vi "Handle Messages.vi"(8 "error in (no error)":errorcluster, 9 "Message Data":variant, 10 "Message":string, 11 "Coffee Shop In":refnum<class "Coffee Shop.lvclass">) -> (0 "error out":errorcluster, 3 "Coffee Shop Out":refnum<class "Coffee Shop.lvclass">)   [LabVIEW 2020, in "Coffee Shop.lvclass"]
uses:
  Coffee Shop.lvclass
  C:/Program Files (x86)/National Instruments/LabVIEW 2020/vi.lib/Astemes/Triarc Framework/Application/Application.lvclass
  C:/Program Files (x86)/National Instruments/LabVIEW 2020/vi.lib/Astemes/Triarc Framework/Process/Process.lvclass
  People/Person/Person.lvclass
  Public/Roles.ctl
  <vilib>/Astemes/Triarc Framework/Process/Process.lvclass/Process.ctl
  <vilib>/Astemes/Triarc Framework/Application/Application.lvclass/Application.ctl
  Coffee Shop.lvclass/Coffee Shop.ctl
  People/Process Job/Job Handler.lvclass
  People/Workers/Cashier/Cashier.lvclass
  C:/Git/astemes-triarc-examples/source/Coffee Shop/Processes/People/Workers/Worker/Worker.lvclass
  People/Customers/Customer/Customer.lvclass
  People/Workers/Barista/Barista.lvclass
  <vilib>/Astemes/Triarc Framework/View/View.lvclass
  <vilib>/Astemes/Triarc Framework/View/View.lvclass/View.ctl
  <vilib>/Astemes/Triarc Framework/Application/Private/Add Process to Map.vi
  <vilib>/Astemes/Triarc Framework/Application/Private/Throw Error If Process Already in App.vi
  <vilib>/Astemes/Triarc Framework/Process/Protected/Messaging/Send Message.vi
  <vilib>/Astemes/Triarc Framework/Process/Public/Lifecycle/Get Lifecycle State.vi
  <vilib>/Astemes/Triarc Framework/Process/Protected/SubVIs/Set Context.vi
  <vilib>/Astemes/Triarc Framework/Process/Stop.vi
  <vilib>/Astemes/Triarc Framework/Application/Private/Remove Process from Map.vi
  <vilib>/Astemes/Triarc Framework/Process/Private/SubVIs/Handle Debug Data.vi
  <vilib>/Astemes/Triarc Framework/Application/Private/Retrieve Process from App.vi
  <vilib>/Astemes/Triarc Framework/Application/Private/Parse Process Name.vi
  <vilib>/Astemes/Triarc Framework/Application/Private/Get Process from Map.vi
  <vilib>/Astemes/Triarc Framework/View/Public/Get View VI Reference.vi
  <vilib>/Utility/error.llb/Clear Errors.vi
  <vilib>/Astemes/Triarc Framework/Process/Public/Lifecycle/Leave Process Loop.vi
  <vilib>/Astemes/Triarc Framework/Process/Private/SubVIs/Wait for finish.vi
  <vilib>/Astemes/Triarc Framework/Process/Private/SubVIs/Set Lifecycle State.vi
  <vilib>/Astemes/Triarc Framework/Logging/Log Debug.vi
  <vilib>/AdvancedString/1D String Array to Delimited String.vi
  <vilib>/Utility/High Resolution Relative Seconds.vi
  <vilib>/Astemes/Triarc Framework/Process/Protected/Messaging/Request Message.vi
  <vilib>/AdvancedString/Delimited String to 1D String Array.vi
  <vilib>/Astemes/Triarc Framework/Process/Private/SubVIs/Enqueue Request Message.vi
  <vilib>/Astemes/Triarc Framework/Application/Application.lvclass
  <vilib>/Utility/error.llb/Error Cluster From Error Code.vi
  <vilib>/Astemes/Triarc Framework/Process/Private/SubVIs/Wait for Response Message.vi
  <vilib>/Astemes/Triarc Framework/Process/Process.lvclass
  People/Workers/Worker/Worker.lvclass
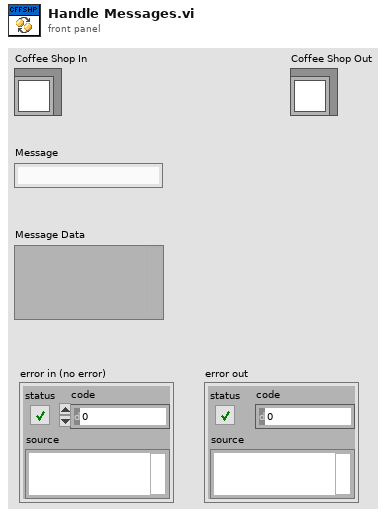
[diagram p1: front panel]
types:
  T1 = typedef "Coffee Shop.lvclass/Roles.ctl" = enum16{"Customer", "Barista", "Cashier"}
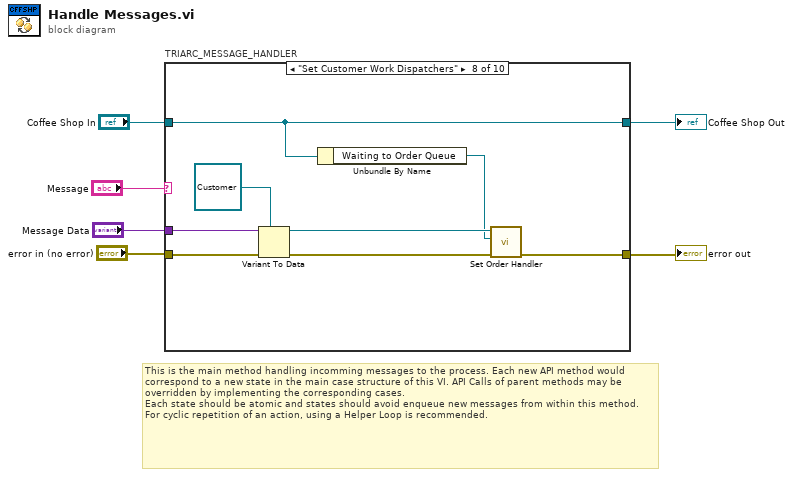
[diagram p0: block diagram]
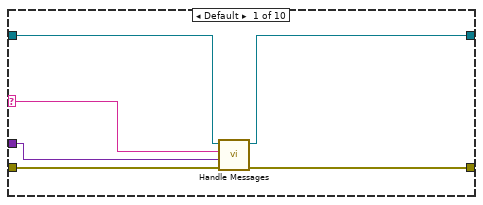
[diagram p2: hidden frame]
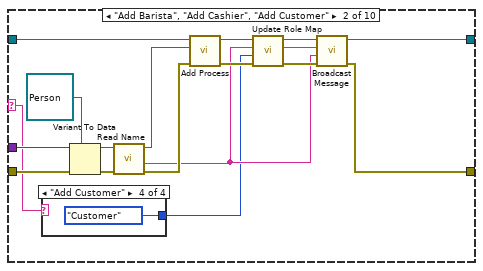
[diagram p3: hidden frame]
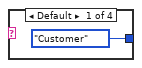
[diagram p4: hidden frame]
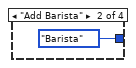
[diagram p5: hidden frame]
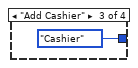
[diagram p6: hidden frame]
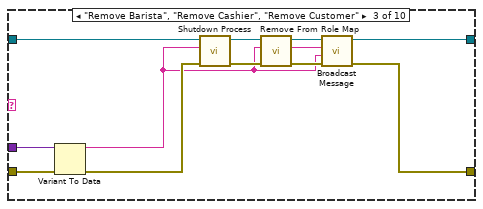
[diagram p7: hidden frame]
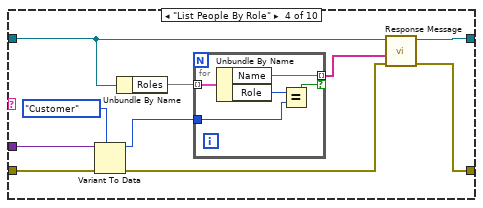
[diagram p8: hidden frame]
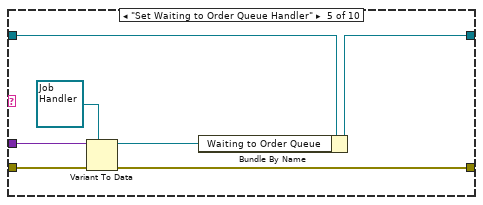
[diagram p9: hidden frame]
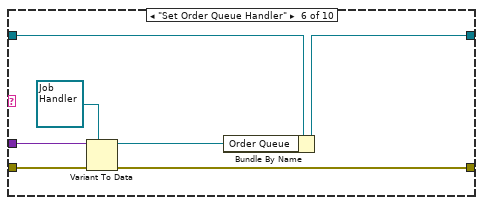
[diagram p10: hidden frame]
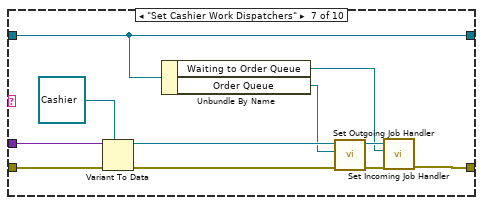
[diagram p11: hidden frame]
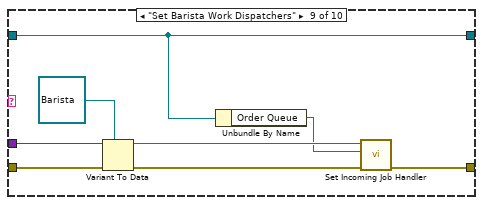
[diagram p12: hidden frame]
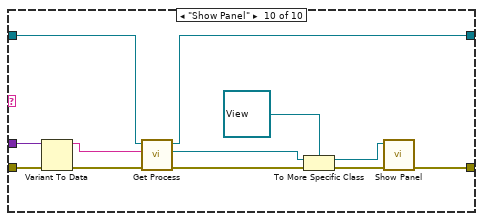
[diagram p13: hidden frame]
diagram:
  # "This is the main method handling incomming messages to the process. Each new API method would correspond to a new state in the main case structure of this VI. API Calls of parent methods may be overridden by implementing the corresponding cases.\nEach state should be atomic and states should avoid enqueue new messages from within this method. For cyclic repetition of an action, using a Helper Loop is recommended."
  n1 = case "TRIARC_MESSAGE_HANDLER" shown="\"Set Customer Work Dispatchers\"" "Message" {
    selector: "Message" -> [w10 w15 _ _ _ _ _ _ _ _]
    tunnel: "error in (no error)" -> [w9 w29 w46 w56 w68 w75 w86 w94 w102 w114]
    tunnel: "Coffee Shop In" -> [w12 w27 w44 w48 w67 w74 w83 w91 w99 w105]
    tunnel: "Message Data" -> [w11 w30 w45 w54 w64 w71 w84 w92 w100 w103]
    tunnel: [w8 w14 w41 w50 w66 w73 w80 w87 w97 w110] -> w2
    tunnel: [w7 w24 w40 w49 w63 w70 w83 w91 w99 w106] -> w1
    frame Default {
      n2 = call-parent "Handle Messages.vi"("error in (no error)"=w9, "Message Data"=w11, "Message"=w10, "Application In"=w12) -> ("error out"=w8:errorcluster, "Application Out"=w7:refnum<class "Coffee Shop.lvclass">)  [unwired: 6 in]
    }
    frame "Add Barista", "Add Cashier", "Add Customer" {
      n3 = case shown="\"Add Customer\"" w15 {
        tunnel: [Roles."Customer" ("Role") Roles."Barista" ("Role") Roles."Cashier" ("Role") Roles."Customer" ("Role")] -> w17
        frame Default {
        }
        frame "Add Barista" {
        }
        frame "Add Cashier" {
        }
        frame "Add Customer" {
        }
      }
      n4 = Variant To Data(error in=w29, type=refnum<class "Person.lvclass"> refnum ("Person.lvclass"), Variant=w30) -> (data=w22:refnum<class "Person.lvclass">, error out=w26:errorcluster)
      n5 = call <vilib>:"Read Name.vi"("error in (no error)"=w26, "Process In"=w22) -> ("error out"=w23:errorcluster, "Name"=w18:string, "Process Out"=w13:refnum<class "Person.lvclass">)  [unwired: 6 in, 1 out]
      n6 = call <vilib>:"Add Process.vi"("error in (no error)"=w23, "Process"=w13, "Application In"=w27) -> ("error out"=w25:errorcluster, "Application Out"=w20:refnum<class "Coffee Shop.lvclass">)  [unwired: 7 in]
      n7 = call "Update Role Map.vi"("error in (no error)"=w25, "Role"=w17, "Name"=w18, "Coffee Shop In"=w20) -> ("error out"=w21:errorcluster, "Result Message"=w16:string, "Coffee Shop Out"=w19:refnum<class "Coffee Shop.lvclass">)  [unwired: 5 in]
      n8 = call-dynamic "Broadcast Message.vi"("error in (no error)"=w21, "Message Data"=w18, "Message"=w16, "Process In"=w19) -> ("error out"=w14:errorcluster, "Process Out"=w24:refnum<class "Coffee Shop.lvclass">)  [unwired: 6 in]
    }
    frame "Remove Barista", "Remove Cashier", "Remove Customer" {
      n9 = Variant To Data(error in=w46, Variant=w45) -> (data=w36:string, error out=w43:errorcluster)  [unwired: 1 in]
      n10 = call <vilib>:"Shutdown Process.vi"("error in (no error)"=w43, "Process Name"=w36, "Application In"=w44) -> ("error out"=w42:errorcluster, "Application Out"=w38:refnum<class "Coffee Shop.lvclass">)  [unwired: 7 in]
      n11 = call "Remove From Role Map.vi"("error in (no error)"=w42, "Name"=w36, "Coffee Shop In"=w38) -> ("error out"=w39:errorcluster, "Result Message"=w35:string, "Coffee Shop Out"=w37:refnum<class "Coffee Shop.lvclass">)  [unwired: 6 in]
      n12 = call-dynamic "Broadcast Message.vi"("error in (no error)"=w39, "Message Data"=w36, "Message"=w35, "Process In"=w37) -> ("error out"=w41:errorcluster, "Process Out"=w40:refnum<class "Coffee Shop.lvclass">)  [unwired: 6 in]
    }
    frame "List People By Role" {
      n13 = Variant To Data(error in=w56, type=Roles."Customer" ("Roles"), Variant=w54) -> (data=w51:T1, error out=w55:errorcluster)
      n14 = Unbundle By Name(w48) -> ("Roles"=w52:map{string, T1})
      n15 = for {
        tunnel: w52 -> [w61] mode=indexing
        tunnel: w51 -> [w57]
        tunnel: [w60] -> w47 mode=indexing if=w59
        n16 = Unbundle By Name(w61) -> ("Name"=w60:string, "Role"=w58:T1)
        n17 = Equal?(x=w58, y=w57) -> (x = y?=w59:bool)
      }
      n18 = call <vilib>:"Response Message.vi"("error in (no error)"=w55, "Response Message Data"=w47, "Process In"=w48) -> ("error out"=w50:errorcluster, "Process Out"=w49:refnum<class "Coffee Shop.lvclass">)  [unwired: 7 in]
    }
    frame "Set Waiting to Order Queue Handler" {
      n19 = Variant To Data(error in=w68, type=refnum<class "Job Handler.lvclass"> refnum ("Job Handler.lvclass"), Variant=w64) -> (data=w62:refnum<class "Job Handler.lvclass">, error out=w66:errorcluster)
      n20 = Bundle By Name(cluster=w67, "Waiting to Order Queue"=w62) -> (w63:refnum<class "Coffee Shop.lvclass">)
    }
    frame "Set Order Queue Handler" {
      n21 = Variant To Data(error in=w75, type=refnum<class "Job Handler.lvclass"> refnum ("Job Handler.lvclass"), Variant=w71) -> (data=w69:refnum<class "Job Handler.lvclass">, error out=w73:errorcluster)
      n22 = Bundle By Name(cluster=w74, "Order Queue"=w69) -> (w70:refnum<class "Coffee Shop.lvclass">)
    }
    frame "Set Cashier Work Dispatchers" {
      n23 = Variant To Data(error in=w86, type=refnum<class "Cashier.lvclass"> refnum ("Cashier.lvclass"), Variant=w84) -> (data=w79:refnum<class "Cashier.lvclass">, error out=w82:errorcluster)
      n24 = Unbundle By Name(w83) -> ("Waiting to Order Queue"=w76:refnum<class "Job Handler.lvclass">, "Order Queue"=w77:refnum<class "Job Handler.lvclass">)
      n25 = call "Set Outgoing Job Handler.vi"("error in (no error)"=w82, "Work Dispatcher"=w77, "Worker In"=w79) -> ("error out"=w81:errorcluster, "Worker Out"=w78:refnum<class "Cashier.lvclass">)  [unwired: 7 in]
      n26 = call "Set Incoming Job Handler.vi"("error in (no error)"=w81, "Job Handler"=w76, "Worker In"=w78) -> ("error out"=w80:errorcluster)  [unwired: 7 in, 1 out]
    }
    frame "Set Customer Work Dispatchers" {
      n27 = Variant To Data(error in=w94, type=refnum<class "Customer.lvclass"> refnum ("Customer.lvclass"), Variant=w92) -> (data=w89:refnum<class "Customer.lvclass">, error out=w90:errorcluster)
      n28 = Unbundle By Name(w91) -> ("Waiting to Order Queue"=w88:refnum<class "Job Handler.lvclass">)
      n29 = call "Set Order Handler.vi"("error in (no error)"=w90, "Order Handler"=w88, "Customer In"=w89) -> ("error out"=w87:errorcluster)  [unwired: 7 in, 1 out]
    }
    frame "Set Barista Work Dispatchers" {
      n30 = Variant To Data(error in=w102, type=refnum<class "Barista.lvclass"> refnum ("Barista.lvclass"), Variant=w100) -> (data=w96:refnum<class "Barista.lvclass">, error out=w98:errorcluster)
      n31 = Unbundle By Name(w99) -> ("Order Queue"=w95:refnum<class "Job Handler.lvclass">)
      n32 = call "Set Incoming Job Handler.vi"("error in (no error)"=w98, "Job Handler"=w95, "Worker In"=w96) -> ("error out"=w97:errorcluster)  [unwired: 7 in, 1 out]
    }
    frame "Show Panel" {
      n33 = Variant To Data(error in=w114, Variant=w103) -> (data=w104:string, error out=w113:errorcluster)  [unwired: 1 in]
      n34 = call <vilib>:"Get Process.vi"("error in (no error)"=w113, "Process Name"=w104, "Application In"=w105) -> ("error out"=w112:errorcluster, "App Process"=w108:refnum<class "Process.lvclass">, "Application Out"=w106:refnum<class "Coffee Shop.lvclass">)  [unwired: 6 in]
      n35 = To More Specific Class(target class=refnum<class "View.lvclass"> refnum ("View Out"), reference=w108, error in=w112) -> (specific class reference=w109:refnum<class "View.lvclass">, error out=w111:errorcluster)
      n36 = call <vilib>:"Show Panel.vi"("error in (no error)"=w111, "View In"=w109) -> ("error out"=w110:errorcluster)  [unwired: 8 in, 1 out]
    }
  }
  "error out" <- w2
  "Coffee Shop Out" <- w1
